vi "uintSquare.vi"(8 "Error in (no error)":errorcluster, 11 "Int in":refnum<class "UintClass.lvclass">) -> (0 "Error out":errorcluster, 1 "Timing":u32, 3 "pow(Int, 2)":refnum<class "UintClass.lvclass">)   [LabVIEW 2011, in "UintClass.lvclass"]
uses:
  UintClass.lvclass
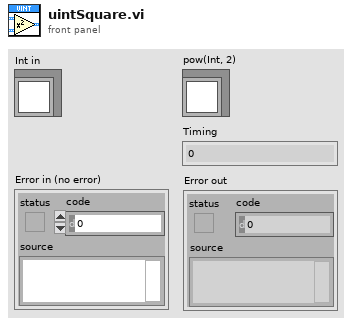
[diagram p1: front panel]
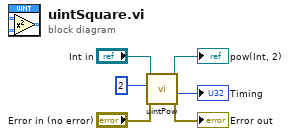
[diagram p0: block diagram]
diagram:
  n1 = call "uintPow.vi"("Error in (no error)"="Error in (no error)", "Exponent"=u32 2, "Int in"="Int in") -> ("Error out"=→"Error out":errorcluster, "Timing"=→"Timing":u32, "pow(Int, Exponent)"=→"pow(Int, 2)":refnum<class "UintClass.lvclass">)  [unwired: 6 in]
